vi "Flatten To String.vi"(8 "error in (no error)":errorcluster, 10 "Variant":variant, 11 "JSON Object Serializer in":refnum<class "Serializer.lvclass">) -> (0 "error out":errorcluster, 2 "String":string, 3 "JSON Object Serializer out":refnum<class "Serializer.lvclass">)   [LabVIEW 2020, in "JKI JSON Object Serialization.lvlib" / "Serializer.lvclass"]
doc: "Converts <b>Variant</b> to JSON formatted <b>String</b>.\n\nGCraftsman JSON Object Serialization Toolkit\nwww.GCraftsman.com\nCopyright (c) 2017, GCraftsman"
uses:
  Serializer.lvclass
  Support/OOP_Utility/Reflection/getObjectPrivateData.vi
  Support/OOP_Utility/Reflection/Assert No Duplicate Named Private Data Elements.vi
  Support/OOP_Utility/Reflection/Assert No Duplicate Named Private Data Elements.vi/91249ab7-5ea3-4d6c-b8df-29db4c9f394f.vi
  Support/OOP_Utility/Reflection/Assert No Duplicate Named Private Data Elements.vi/f7c1a62c-1232-4a35-ba9e-0fa75d385864.vi
  <vilib>/AdvancedString/1D String Array to Delimited String.vi
  <vilib>/dlg_ctls.llb/Space Constant.vi
  Support/OOP_Utility/Reflection/Assert No Duplicate Named Private Data Elements.vi/91249ab7-5ea3-4d6c-b8df-29db4c9f394f.vi/73eff78f-802f-4e82-99e6-5ec6d44c8b1c.vi
  Support/OOP_Utility/Reflection/Assert No Duplicate Named Private Data Elements.vi/91249ab7-5ea3-4d6c-b8df-29db4c9f394f.vi/a79ef678-9021-4176-8e9d-ef71acec083e.vi
  Support/OOP_Utility/Reflection/Assert No Duplicate Named Private Data Elements.vi/91249ab7-5ea3-4d6c-b8df-29db4c9f394f.vi/6194b64b-8f19-4369-9ca4-18e99c56e175.vi
  Support/OOP_Utility/Reflection/Assert No Duplicate Named Private Data Elements.vi/91249ab7-5ea3-4d6c-b8df-29db4c9f394f.vi/4000f349-3ba7-45cd-93a4-b1a8967d5605.vi
  <vilib>/Utility/LVClass/Get LV Class Name.vi
  Support/OOP_Utility/Reflection/reflectionPool.vi
  <userlib>/_OpenG.lib/lvdata/lvdata.llb/Get Cluster Element Names__ogtk.vi
  <vilib>/Utility/error.llb/Error Cluster From Error Code.vi
  <userlib>/_OpenG.lib/lvdata/lvdata.llb/Cluster to Array of VData__ogtk.vi
  <userlib>/_OpenG.lib/lvdata/lvdata.llb/Set Data Name__ogtk.vi
  <userlib>/_OpenG.lib/lvdata/lvdata.llb/Array of VData to VCluster__ogtk.vi
  <vilib>/addons/_JKI.lib/Serialization/JSON/Serializer/JSON Serializer/JSON Serializer.lvclass
  Serializer.lvclass/Serializer.ctl
  Support/OOP_Utility/OOP_Utility.lvlib
  <vilib>/Utility/Data Type/NI_Data Type.lvlib
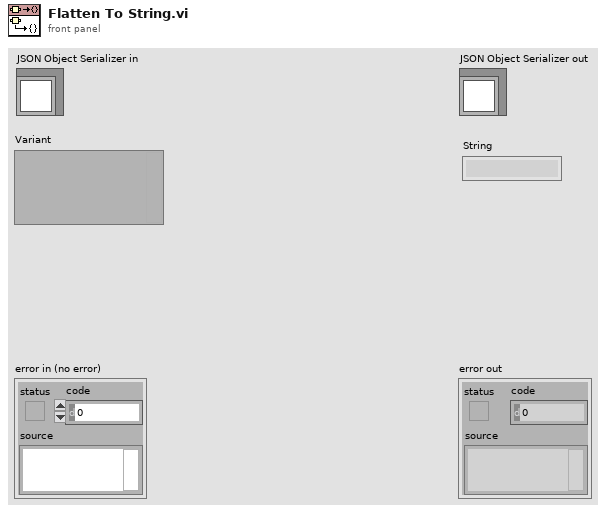
[diagram p1: front panel]
types:
  T1 = typedef "NI_Data Type.lvlib/Data Type.ctl" = enum8{"Invalid Type", "Void", "I8", "I16", "I32", "I64", "U8", "U16", "U32", "U64", "Single Float", "Double Float", "Extended Float", "Single Complex", "Double Complex", "Extended Complex", "Enum U8", "Enum U16", "Enum U32", "Enum U64", "Single Float With Unit", "Double Float With Unit", "Extended Float With Unit", "Single Complex with Unit", "Double Complex with Unit", "Extended Complex with Unit", "Boolean", "String", "Path", "Picture", "Tag", "Array", "Cluster", "Variant", "LV Variant", "Waveform", "Timestamp", "Digital Waveform", "Digital Data", "ExpressData", "Refnum", "External Data", "VI", "Poly VI", "LabVIEW Class Instance", "Fixed Point", "Set Collection", "Map Collection"}
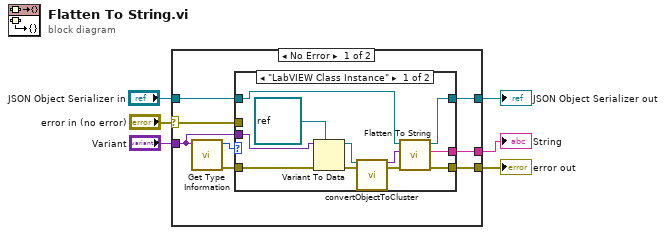
[diagram p0: block diagram]
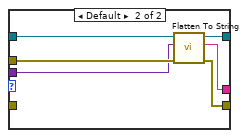
[diagram p2: hidden frame]
diagram:
  n1 = case shown="No Error" "error in (no error)" {
    selector: "error in (no error)" -> [w10 w32]
    tunnel: [w14 w32] -> w6
    tunnel: [w13 _] -> w5
    tunnel: [w12 w33] -> w4
    tunnel: "Variant" -> [w9 _]
    tunnel: "JSON Object Serializer in" -> [w11 w33]
    frame No Error {
      n2 = call <vilib>:"Get Type Information.vi"("variant"=w9) -> ("error out"=w7:errorcluster, "type"=w8:T1)  [unwired: 6 in, 3 out]
      n3 = case shown="\"LabVIEW Class Instance\"" w8 {
        tunnel: [w17 w31] -> w14
        tunnel: [w18 w30] -> w13
        tunnel: [w19 w29] -> w12
        tunnel: w10 -> [_ w28]
        tunnel: w9 -> [w25 w27]
        tunnel: w11 -> [w20 w26]
        tunnel: w7 -> [w23 _]
        frame "LabVIEW Class Instance" {
          n4 = Variant To Data(error in=w23, type=refnum<class> refnum ("LabVIEW Object"), Variant=w25) -> (data=w22:refnum<class>, error out=w21:errorcluster)
          n5 = call "convertObjectToCluster.vi"("Object in"=w22, "error in"=w21) -> ("VCluster"=w15:variant, "error out"=w16:errorcluster)  [unwired: 16 in]
          n6 = call-parent "Flatten To String.vi"("error in (no error)"=w16, "Variant"=w15, "JSON Serializer in"=w20) -> ("error out"=w17:errorcluster, "String"=w18:string, "JSON Serializer out"=w19:refnum<class "Serializer.lvclass">)  [unwired: 6 in]
        }
        frame Default {
          n7 = call-parent "Flatten To String.vi"("error in (no error)"=w28, "Variant"=w27, "JSON Serializer in"=w26) -> ("error out"=w31:errorcluster, "String"=w30:string, "JSON Serializer out"=w29:refnum<class "Serializer.lvclass">)  [unwired: 6 in]
        }
      }
    }
    frame Error {
    }
  }
  "error out" <- w6
  "JSON Object Serializer out" <- w4
  "String" <- w5
